vi "Read np.vi"(8 "error in (no error)":errorcluster, 11 "RotatorTracking in":refnum<class "RotatorTracking.lvclass">) -> (0 "error out":errorcluster, 2 "np":dbl[unit] min=0.0 max=6.283185307179586, 3 "RotatorTracking out":refnum<class "RotatorTracking.lvclass">)   [LabVIEW 2022 SP3, in "TCSDataDefinitions.lvlib" / "TCSMountControlStatus.lvlib" / "RotatorTracking.lvclass"]
uses:
  RotatorTracking.lvclass
  RotatorTracking.lvclass/RotatorTracking.ctl
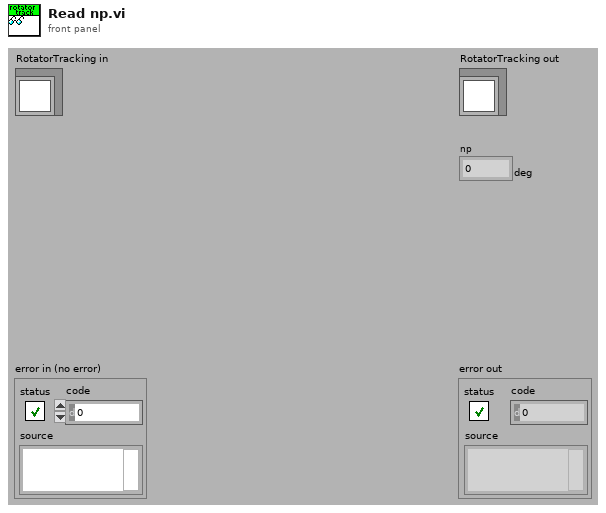
[diagram p1: front panel]
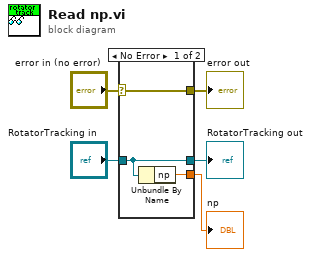
[diagram p0: block diagram]
diagram:
  n1 = case shown="No Error" "error in (no error)" {
    selector: "error in (no error)" -> [w8 w9]
    tunnel: [w8 w9] -> w4
    tunnel: [w7 w10] -> w2
    tunnel: "RotatorTracking in" -> [w7 w10]
    tunnel: [w6 _] -> w1
    frame No Error {
      n2 = Unbundle By Name(w7) -> ("np"=w6:dbl[unit])
    }
    frame Error {
    }
  }
  "error out" <- w4
  "RotatorTracking out" <- w2
  "np" <- w1
